vi "musk_AEB.vi"(1 "x,y 배열":cluster{"x":dbl, "y":dbl}[](array[cluster])) -> (0 "AEB!!":bool)   [LabVIEW 2015]
panel:
  # "2200"
  # "-1000"
  # "1000"
  # "2200"
  # "-1000"
  # "1000"
  # "-1000"
  # "1000"
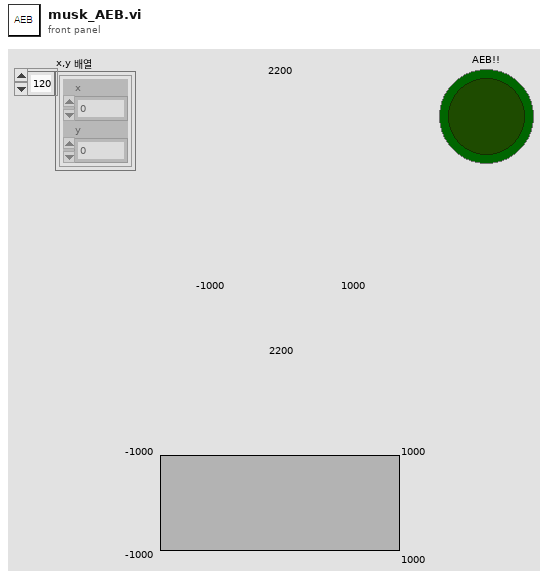
[diagram p1: front panel]
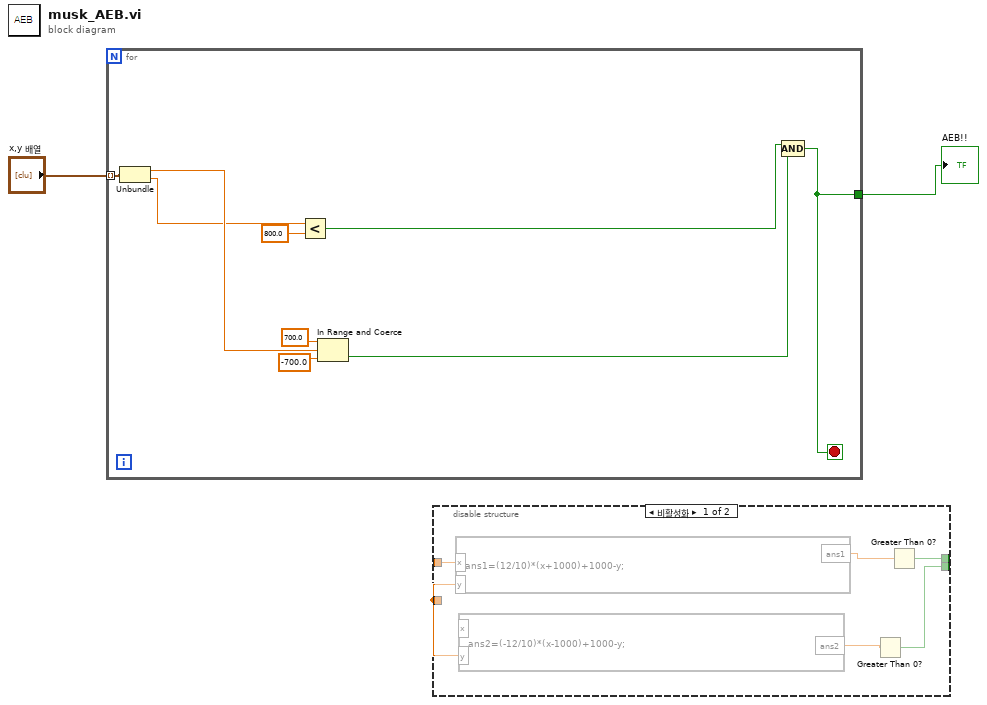
[diagram p0: block diagram]
diagram:
  n1 = for {
    tunnel: "x,y 배열" -> [w11] mode=indexing
    tunnel: [w10] -> w2
    stop <- w10 stop-if-true
    n2 = Unbundle(w11) -> ("x"=w9:dbl, "y"=w5:dbl)
    n3 = Less?(x=w5, y=800.0) -> (x < y?=w3:bool)
    n4 = In Range and Coerce(upper limit=700.0 ("상위 리미트"), x=w9, lower limit=-700.0 ("하위 리미트")) -> (In Range?=w6:bool)  [unwired: 1 out]
    n5 = Compound Arithmetic op=AND ("복합 연산")(w3, w6) -> (w10:bool)
  }
  "AEB!!" <- w2
  n6 = disable-structure shown="비활성화" {
    disable-tunnel: [w16 _] -> _
    disable-tunnel: _ -> [w15 _]
    disable-tunnel: [w13 _] -> _
    disable-tunnel: _ -> [w12 _]
    frame Disabled {
      n7 = formula code="ans1=(12/10)*(x+1000)+1000-y;"("x"=w12, "y"=w15) -> ("ans1"=w17:dbl)
      n8 = formula code="ans2=(-12/10)*(x-1000)+1000-y;"("y"=w15) -> ("ans2"=w14:dbl)  [unwired: 1 in]
      n9 = Greater Than 0?(x=w14) -> (x > 0?=w13:bool)
      n10 = Greater Than 0?(x=w17) -> (x > 0?=w16:bool)
    }
    frame Enabled {
    }
  }
